vi "FTW-CodeGen-Prototype.vi"(0 "REPLACE_SQLite Connection":refnum<data-value>, 2 "REPLACE_SQL Script":string, 5 "ADAPT_Row Datatype":cluster{"Column":variant}, 11 "REPLACE_error in":errorcluster) -> (4 "REPLACE_SQLite Connection out":refnum<data-value>, 6 "ADAPT_Result Set":cluster{"Column":variant}[](array[cluster]), 8 "REPLACE_SQL Debug String":string, 15 "REPLACE_error out":errorcluster)   [LabVIEW 2015, in "FTW-SQLite-Fetch.xnode"]
uses:
  FTW-SQLite-Fetch.xnode
  src/database/core/FTW-SQLite-Core-Structure.ctl
  src/error/FTW-ERR-ThrowError.vi
  src/error/FTW-ERR-CallChain.vi
  src/error/FTW-ERR-NoErrorConstant.vi
  src/string/FTW-STR-ReplaceWhitespace.vi
  src/string/FTW-STR-Array-Delimit.vi
  src/error/FTW-ERR-Clear.vi
  src/regex/FTW-Regex-ReplaceAll.vi
panel:
  # "Inputs"
  # "Outputs"
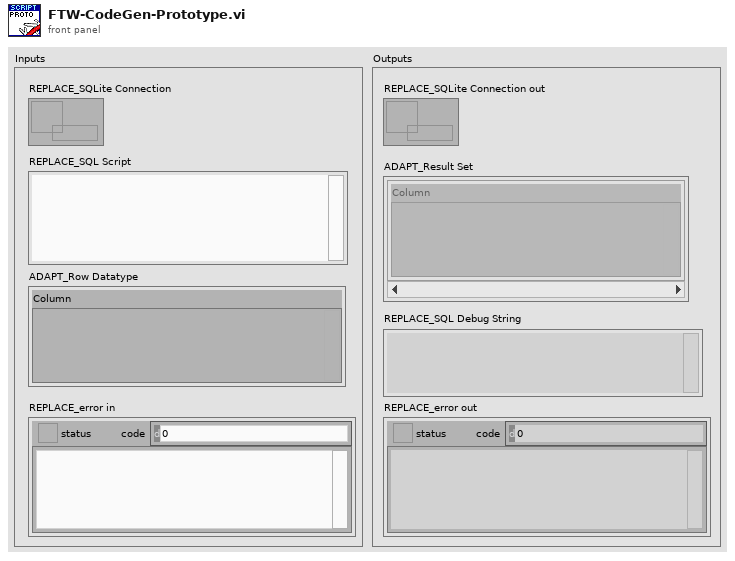
[diagram p1: front panel]
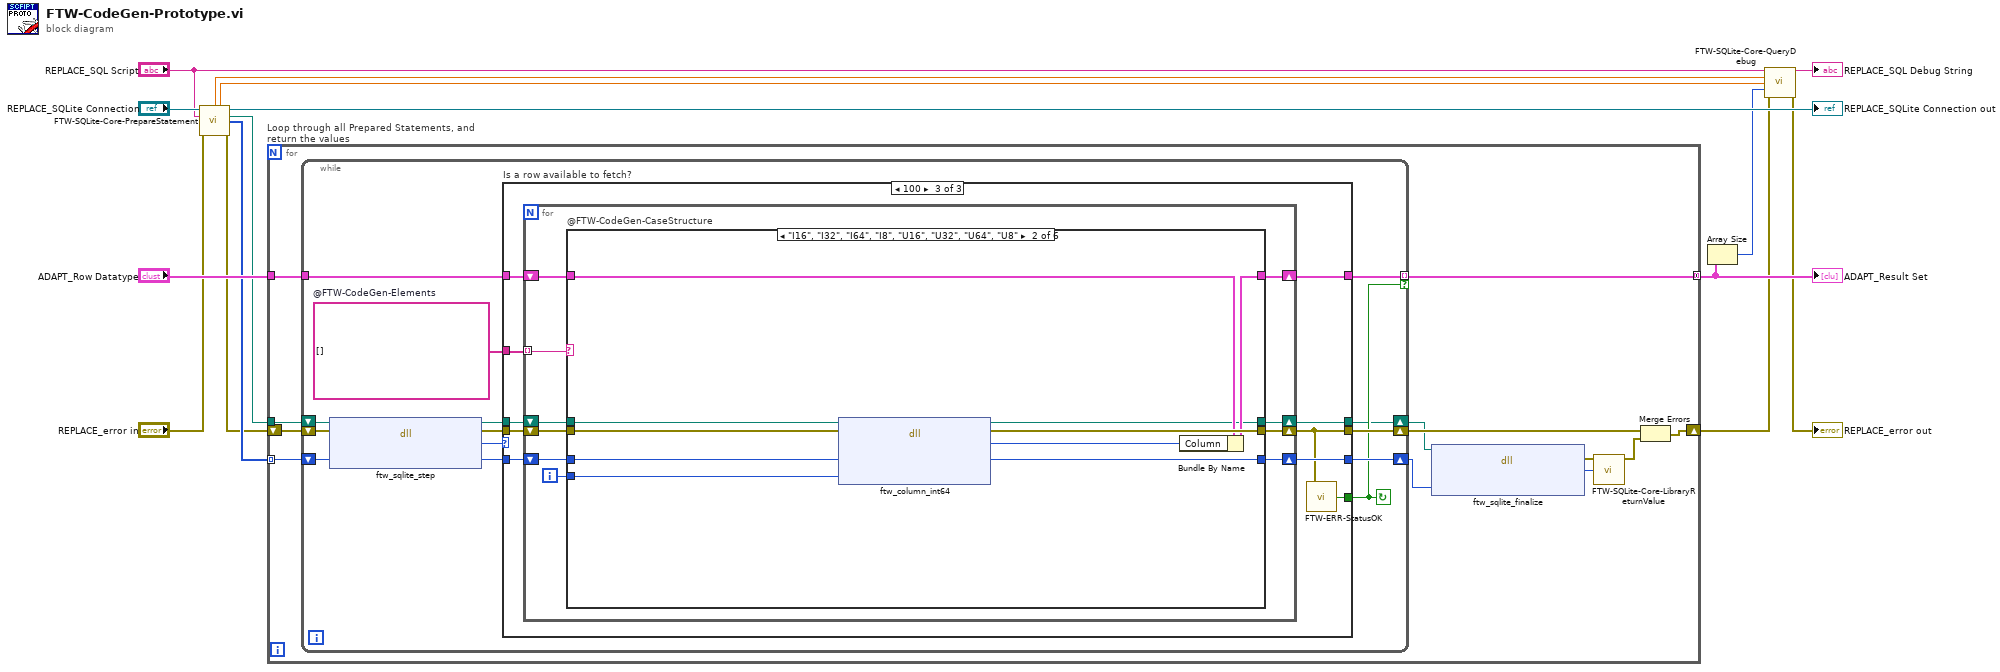
[diagram p0: block diagram]
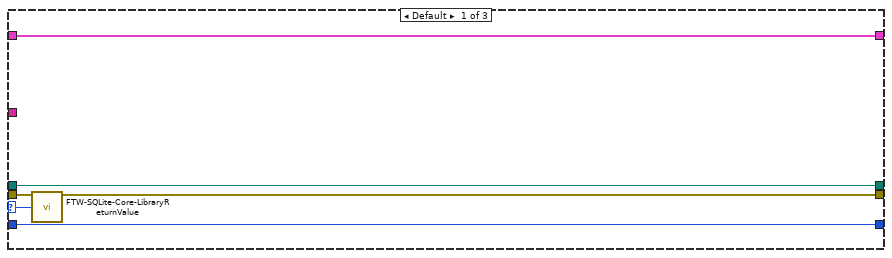
[diagram p2: hidden frame]
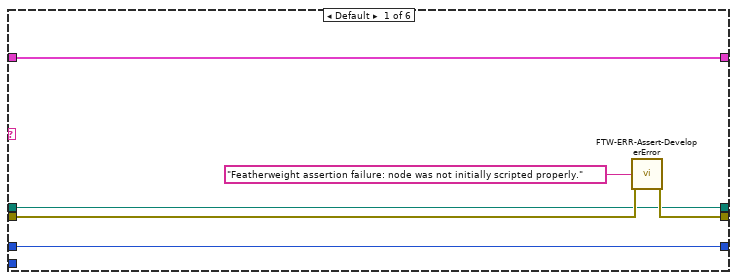
[diagram p4: hidden frame]
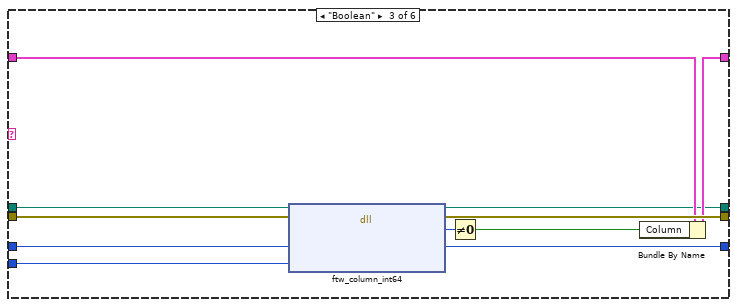
[diagram p5: hidden frame]
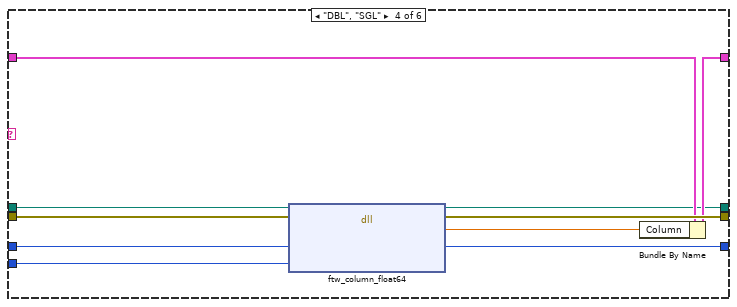
[diagram p6: hidden frame]
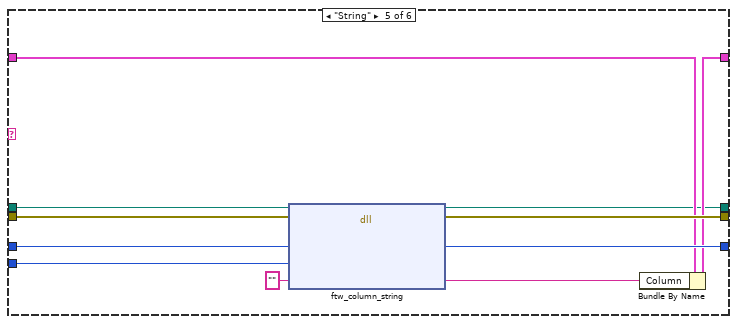
[diagram p7: hidden frame]
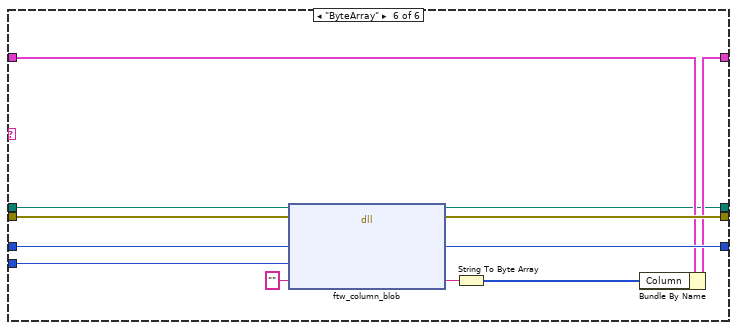
[diagram p8: hidden frame]
diagram:
  n1 = call "FTW-SQLite-Core-PrepareStatement.vi"("SQLite Connection"="REPLACE_SQLite Connection", "SQL Statement"="REPLACE_SQL Script", "error in"="REPLACE_error in") -> ("Begin Timestamp"=w3:dbl, "Compile Time"=w2:dbl, "SQLite Connection out"=→"REPLACE_SQLite Connection out":refnum<data-value>, "Library Filepath"=w1:path, "Prepared Statements"=w11:i64[], "error out"=w5:errorcluster)  [unwired: 7 in]
  n2 = for "Loop through all Prepared Statements, and return the values" {
    tunnel: w11 -> [w19] mode=indexing
    shift-right: [w25] -> w4
    shift-left: w5 -> [w20]
    tunnel: "ADAPT_Row Datatype" -> [w21]
    tunnel: [w18] -> w12 mode=concatenating
    tunnel: w1 -> [w16]
    n3 = while {
      shift-right: [w36] -> w23
      shift-left: w20 -> [w41]
      shift-right: [w35] -> w22
      shift-left: w19 -> [w40]
      tunnel: w21 -> [w32]
      tunnel: [w34] -> w18 mode=indexing if=w33
      shift-right: [w29] -> w17
      shift-left: w16 -> [w28]
      stop <- w33 continue-if-true
      w31 = string[] []  # @FTW-CodeGen-Elements
      n4 = dll-call lib="?" fn="ftw_sqlite_step"(path in=w28, error in=w41, "Prepared Statement Pointer"=w40) -> (path out=w30:path, error out=w38:errorcluster, "Return Value"=w39:i32, "Prepared Statement Pointer"=w37:i64)  [unwired: 1 in]
      n5 = case "Is a row available to fetch?" shown="100" w39 {
        selector: w39 -> [w47 _ _]
        tunnel: w38 -> [w46 w51 w61]
        tunnel: w37 -> [w44 w50 w60]
        tunnel: [w45 w51 w57] -> w36
        tunnel: [w44 w50 w59] -> w35
        tunnel: w32 -> [w43 w49 w56]
        tunnel: [_ _ w58] -> w33
        tunnel: [w43 w49 w55] -> w34
        tunnel: w31 -> [_ _ w54]
        tunnel: w30 -> [w42 w48 w53]
        tunnel: [w42 w48 w52] -> w29
        frame Default {
          n6 = call "FTW-SQLite-Core-LibraryReturnValue.vi"("error in"=w46, "Return Value"=w47) -> ("error out"=w45:errorcluster)  [unwired: 13 in]
        }
        frame 101 {
          # "SQLITE_DONE=101 -- looks like there are no more columns to fetch!"
        }
        frame 100 {
          n7 = for {
            shift-right: [w68] -> w57
            shift-left: w61 -> [w71]
            shift-right: [w69] -> w59
            shift-left: w60 -> [w70]
            shift-right: [w66] -> w55
            shift-left: w56 -> [w67]
            tunnel: w54 -> [w64] mode=indexing
            shift-right: [w62] -> w52
            shift-left: w53 -> [w63]
            i -> [w65]
            n8 = case "@FTW-CodeGen-CaseStructure" shown="\"I16\", \"I32\", \"I64\", \"I8\", \"U16\", \"U32\", \"U64\", \"U8\"" w64 {
              tunnel: w71 -> [w75 w85 w96 w106 w117 w129]
              tunnel: w70 -> [w77 w84 w95 w105 w116 w128]
              tunnel: [w77 w87 w98 w108 w119 w131] -> w69
              tunnel: [w74 w86 w97 w107 w118 w130] -> w68
              tunnel: w67 -> [w76 w82 w93 w103 w114 w126]
              tunnel: [w76 w81 w92 w102 w113 w125] -> w66
              tunnel: w65 -> [_ w83 w94 w104 w115 w127]
              tunnel: w63 -> [w72 w79 w89 w100 w110 w121]
              tunnel: [w72 w78 w88 w99 w109 w120] -> w62
              frame Default {
                n9 = call "FTW-ERR-Assert-DeveloperError.vi"("Reason this error should never happen"="Featherweight assertion failure: node was not initially scripted properly.", "error in"=w75) -> ("error out"=w74:errorcluster)  [unwired: 13 in]
              }
              frame "I16", "I32", "I64", "I8", "U16", "U32", "U64", "U8" {
                n10 = dll-call lib="?" fn="ftw_column_int64"(path in=w79, error in=w85, "Prepared Statement Pointer"=w84, "Column Index"=w83) -> (path out=w78:path, error out=w86:errorcluster, "I64 Value"=w80:i64, "Prepared Statement Pointer"=w87:i64)  [unwired: 2 in]
                n11 = Bundle By Name(cluster=w82, "Column"=w80) -> (w81:cluster{"Column":variant})
              }
              frame "Boolean" {
                n12 = dll-call lib="?" fn="ftw_column_int64"(path in=w89, error in=w96, "Prepared Statement Pointer"=w95, "Column Index"=w94) -> (path out=w88:path, error out=w97:errorcluster, "I64 Value"=w91:i64, "Prepared Statement Pointer"=w98:i64)  [unwired: 2 in]
                n13 = Not Equal To 0?(x=w91) -> (x != 0?=w90:bool)
                n14 = Bundle By Name(cluster=w93, "Column"=w90) -> (w92:cluster{"Column":variant})
              }
              frame "DBL", "SGL" {
                n15 = dll-call lib="?" fn="ftw_column_float64"(path in=w100, error in=w106, "Prepared Statement Pointer"=w105, "Column Index"=w104) -> (path out=w99:path, error out=w107:errorcluster, "DBL Value"=w101:dbl, "Prepared Statement Pointer"=w108:i64)  [unwired: 2 in]
                n16 = Bundle By Name(cluster=w103, "Column"=w101) -> (w102:cluster{"Column":variant})
              }
              frame "String" {
                n17 = dll-call lib="?" fn="ftw_column_string"(path in=w110, error in=w117, "Prepared Statement Pointer"=w116, "Column Index"=w115, "String Value"="") -> (path out=w109:path, error out=w118:errorcluster, "Prepared Statement Pointer"=w119:i64, "String Value"=w112:string)  [unwired: 3 in]
                n18 = Bundle By Name(cluster=w114, "Column"=w112) -> (w113:cluster{"Column":variant})
              }
              frame "ByteArray" {
                n19 = dll-call lib="?" fn="ftw_column_blob"(path in=w121, error in=w129, "Prepared Statement Pointer"=w128, "Column Index"=w127, "String Value"="") -> (path out=w120:path, error out=w130:errorcluster, "Prepared Statement Pointer"=w131:i64, "String Value"=w124:string)  [unwired: 3 in]
                n20 = String To Byte Array(string=w124) -> (unsigned byte array=w122:u8[])
                n21 = Bundle By Name(cluster=w126, "Column"=w122) -> (w125:cluster{"Column":variant})
              }
            }
          }
          n22 = call "FTW-ERR-StatusOK.vi"("error to check"=w57) -> ("Status OK?"=w58:bool)
        }
      }
    }
    n23 = dll-call lib="?" fn="ftw_sqlite_finalize"(path in=w17, "Prepared Statement Pointer"=w22) -> (error out=w27:errorcluster, "Return Value"=w26:i32)  [unwired: 3 in, 1 out]
    n24 = call "FTW-SQLite-Core-LibraryReturnValue.vi"("error in"=w27, "Return Value"=w26) -> ("error out"=w24:errorcluster)  [unwired: 13 in]
    n25 = Merge Errors(w23, w24) -> (w25:errorcluster)
  }
  "ADAPT_Result Set" <- w12
  n26 = Array Size(array=w12) -> (size(s)=w9:i32)
  n27 = call "FTW-SQLite-Core-QueryDebug.vi"("SQL Script"="REPLACE_SQL Script", "Begin Timestamp"=w3, "Compile Time"=w2, "Rows Affected"=w9, "error in"=w4) -> ("SQL Debug String"=→"REPLACE_SQL Debug String":string, "error out"=→"REPLACE_error out":errorcluster)  [unwired: 9 in]
